vi "_FPGA_Aux_DigitalPulses.vi"(6 "Cycle in":u64, 7 "reset":bool, 8 "TargetCycle2(i,f)":u64, 9 "AuxVoltage2":i16, 10 "TargetCycle1(i,f)":u64, 11 "AuxVoltage1":i16) -> (2 "AuxVoltage":fxp<+/-,16,14>)   [LabVIEW 2018]
uses:
  <instrlib>/_niInstr/Basic Elements/v1/FPGA/niInstr Basic Elements v1 FPGA.lvlib
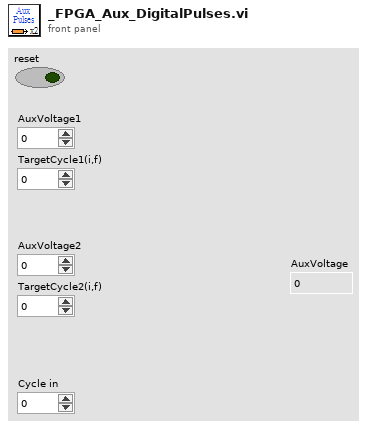
[diagram p1: front panel]
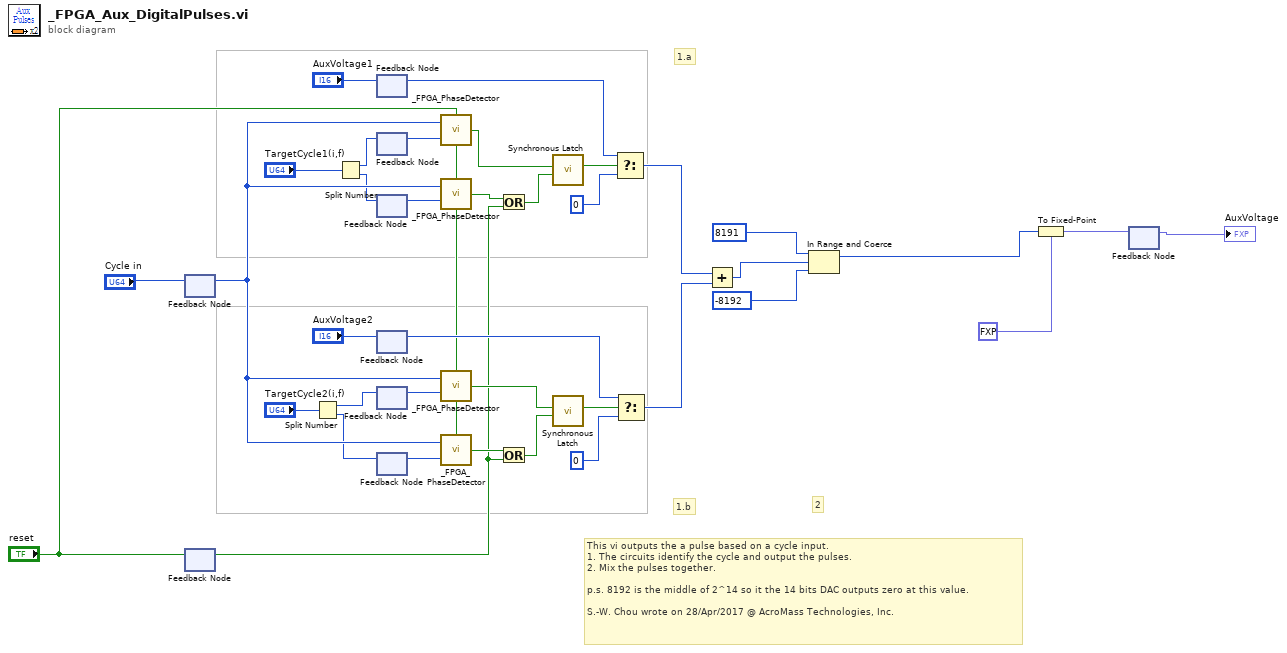
[diagram p0: block diagram]
diagram:
  # "2"
  # "1.b"
  # "1.a"
  # "This vi outputs the a pulse based on a cycle input.\n1. The circuits identify the cycle and output the pulses.\n2. Mix the pulses together. \n\np.s. 8192 is the middle of 2^14 so it the 14 bits DAC outputs zero at this value.\n\nS.-W. Chou wrote on 28/Apr/2017 @ AcroMass Technologies, Inc."
  n1 = feedback #1() -> (w29:u64)  [unwired: 1 in]
  n2 = feedback-in #1("Cycle in") -> ()
  n3 = feedback-in #2("reset") -> ()
  n4 = feedback #2() -> (w4:bool)  [unwired: 1 in]
  n5 = Split Number(x="TargetCycle2(i,f)") -> (hi(x)=w11:u32, lo(x)=w10:u32)
  n6 = Split Number(x="TargetCycle1(i,f)") -> (hi(x)=w14:u32, lo(x)=w13:u32)
  n7 = feedback #3() -> (w22:i16)  [unwired: 1 in]
  n8 = feedback-in #3("AuxVoltage1") -> ()
  n9 = feedback #4() -> (w33:u32)  [unwired: 1 in]
  n10 = feedback-in #4(w14) -> ()
  n11 = feedback #5() -> (w12:u32)  [unwired: 1 in]
  n12 = feedback-in #5(w13) -> ()
  n13 = feedback #6() -> (w20:i16)  [unwired: 1 in]
  n14 = feedback-in #6("AuxVoltage2") -> ()
  n15 = feedback #7() -> (w31:u32)  [unwired: 1 in]
  n16 = feedback-in #7(w11) -> ()
  n17 = feedback #8() -> (w28:u32)  [unwired: 1 in]
  n18 = feedback-in #8(w10) -> ()
  n19 = call "_FPGA_PhaseDetector.vi"("Reset"="reset", "Target"=w33, "Cycle in"=w29) -> ("strobe out"=w27:bool)
  n20 = call "_FPGA_PhaseDetector.vi"("Reset"="reset", "Target"=w12, "Cycle in"=w29) -> ("strobe out"=w26:bool)
  n21 = call "_FPGA_PhaseDetector.vi"("Reset"="reset", "Target"=w31, "Cycle in"=w29) -> ("strobe out"=w25:bool)
  n22 = call "_FPGA_PhaseDetector.vi"("Reset"="reset", "Target"=w28, "Cycle in"=w29) -> ("strobe out"=w24:bool)
  n23 = Or(x=w26, y=w4) -> (x .or. y?=w6:bool)
  n24 = Or(x=w24, y=w4) -> (x .or. y?=w5:bool)
  n25 = call <instrlib>:"Synchronous Latch.vi"("clear"=w6, "set"=w27) -> ("out"=w23:bool)  [unwired: 9 in]
  n26 = call <instrlib>:"Synchronous Latch.vi"("clear"=w5, "set"=w25) -> ("out"=w21:bool)  [unwired: 9 in]
  n27 = Select(t=w22, s=w23, f=i16 0) -> (s? t:f=w17:i16)
  n28 = Select(t=w20, s=w21, f=i16 0) -> (s? t:f=w16:i16)
  n29 = Add(x=w17, y=w16) -> (x+y=w9:i16)
  n30 = In Range and Coerce(upper limit=i16 8191 ("f"), x=w9, lower limit=i16 -8192 ("f")) -> (coerced(x)=w2:i16)  [unwired: 1 out]
  n31 = To Fixed-Point(fixed-point type=fxp<+/-,16,14> 0.0, number=w2) -> (fixed-point=w37:fxp<+/-,16,14>)
  n32 = feedback #9() -> (→"AuxVoltage":fxp<+/-,16,14>)  [unwired: 1 in]
  n33 = feedback-in #9(w37) -> ()
